vi "Lab Panel V5.24.1.vi"() -> ()   [LabVIEW 2013] (continued)
                n852 = local write "run lab04-1"(w1517) -> ()
                n853 = case shown="True" w1517 {
                  tunnel: w1523 -> [_ w1561]
                  tunnel: w1522 -> [_ w1560]
                  tunnel: w1520 -> [w1525 w1559]
                  tunnel: w1521 -> [_ w1558]
                  tunnel: w1519 -> [_ w1557]
                  tunnel: [w1524 w1556] -> w1518
                  tunnel: w1516 -> [_ w1555]
                  tunnel: w1515 -> [_ w1554]
                  tunnel: w1514 -> [_ w1553]
                  tunnel: w1513 -> [_ w1551]
                  frame False {
                    # "stop test"
                    n854 = stacked-sequence {
                      tunnel: w1525 -> [w1534 _]
                      tunnel: [w1526 _] -> w1524
                      frame #0 {
                        n855 = local read "DISP LAB04-1"() -> (w1533:T4)
                        n856 = Unbundle(w1533) -> ("CYCLE"=w1531:dbl, "MINS"=w1532:dbl)  [unwired: 1 out]
                        n857 = case shown="\"CYCLE TEST\"" w1534 {
                          tunnel: w1532 -> [_ _ w1541]
                          tunnel: w1531 -> [w1539 w1540 _]
                          tunnel: [w1539 w1540 w1541] -> w1530
                          frame "CHART TEST", Default {
                          }
                          frame "CYCLE TEST" {
                          }
                          frame "T-RISE TEST" {
                          }
                        }
                        n858 = local read "TDMS LAB04-1"() -> (w1538:refnum<k34>)
                        n859 = Build Array("STOPPED") -> (w1535:string[])
                        n860 = Build Array(w1530) -> (w1529:dbl[])
                        n861 = TDMS Write(0:w1538, 5:"TEST RESULT", 7:w1535, 9:w1529) -> (4:w1527:refnum<k34>, 15:w1528:errorcluster)  [unwired: 2 in, 2 out]
                        n862 = TDMS Close(8:w1528, 11:w1527) -> (0:w1526:errorcluster)  [unwired: 1 out]
                      }
                      frame #1 {
                        n863 = local read "DISP LAB04-1"() -> (w1545:T4)
                        n864 = stacked-sequence {
                          tunnel: "LAB04-1" -> [w1547 w1549]
                          frame #0 {
                            n865 = call "sub vi - defrag tdms v1.vi"("panel id"=w1547) -> ("error out"=w1546:errorcluster)  [unwired: 10 in]
                            n866 = local write "data file error"(w1546) -> ()
                          }
                          frame #1 {
                            n867 = call "Save data file (stop) v3.vi"("panel id"=w1549) -> ("network file save error"=w1548:errorcluster)  [unwired: 9 in, 1 out]
                            n868 = local write "RESULT LAB04-1"(FALSE) -> ()
                            n869 = local write "data file error"(w1548) -> ()
                          }
                        }
                        n870 = Bundle(cluster=w1545, "STATUS"="STOP") -> (w1543:T4)  [unwired: 2 in]
                        n871 = local write "DISP LAB04-1"(w1543) -> ()
                      }
                    }
                  }
                  frame True {
                    n872 = local read "SIG LAB04-1"() -> (w1552:T2)
                    n873 = stacked-sequence {
                      seq-local: [w1563 _] -> [_ w1567]
                      tunnel: w1561 -> [_ w1577]
                      tunnel: w1560 -> [_ w1576]
                      tunnel: w1559 -> [_ w1575]
                      tunnel: w1558 -> [_ w1574]
                      tunnel: w1557 -> [_ w1573]
                      tunnel: [_ w1572] -> w1556
                      tunnel: w1555 -> [_ w1571]
                      tunnel: w1554 -> [_ w1570]
                      tunnel: w1553 -> [_ w1569]
                      tunnel: w1552 -> [w1562 w1568]
                      tunnel: w1551 -> [_ w1566]
                      frame #0 {
                        n874 = Unbundle(w1562) -> ("AMPS"=w1565:dbl)  [unwired: 4 out]
                        n875 = call "Check For Amps on v1.vi"("ID"="LAB04-1", "amps"=w1565) -> ("amps"=w1563:bool)  [unwired: 9 in]
                      }
                      frame #1 {
                        n876 = case shown="True" w1567 {
                          tunnel: w1577 -> [_ w1590]
                          tunnel: w1576 -> [_ w1589]
                          tunnel: w1575 -> [_ w1588]
                          tunnel: w1574 -> [_ w1587]
                          tunnel: w1573 -> [_ w1586]
                          tunnel: [errorcluster {"status"=FALSE, "code"=0, "source"=""} ("error out") w1585] -> w1572
                          tunnel: w1571 -> [_ w1584]
                          tunnel: w1570 -> [_ w1583]
                          tunnel: w1569 -> [_ w1582]
                          tunnel: w1568 -> [_ w1581]
                          tunnel: w1566 -> [_ w1580]
                          frame False {
                            w1578 = FALSE
                            n877 = local write "RUN LAB04-1"(w1578) -> ()
                            n878 = local write "run lab04-1"(w1578) -> ()
                          }
                          frame True {
                            n879 = stacked-sequence {
                              seq-local: [w1591 _ _ _ _] -> [_ w1615 _ _ _]
                              tunnel: w1590 -> [w1596 _ _ _ _]
                              tunnel: w1589 -> [w1592 _ _ _ _]
                              tunnel: w1588 -> [w1606 _ _ _ _]
                              tunnel: w1587 -> [w1599 _ _ _ _]
                              tunnel: w1586 -> [w1594 _ _ _ _]
                              tunnel: [_ w1610 _ _ _] -> w1585
                              tunnel: w1584 -> [_ _ _ w1636 _]
                              tunnel: w1583 -> [_ _ _ w1635 _]
                              tunnel: w1582 -> [_ _ _ w1634 _]
                              tunnel: w1581 -> [_ _ _ _ _]
                              tunnel: w1580 -> [_ _ _ _ w1650]
                              frame #0 {
                                w1593 = "\\"
                                n880 = local read "SET LAB04-1"() -> (w1601:T5)
                                n881 = case shown="\"CYCLE TEST\"" w1606 {
                                tunnel: ["L04-1-CHART TEST-" "L04-1-CYCLE TEST-" "L04-1-T-RISE TEST-"] -> w1602
                                frame "CHART TEST", Default {
                                }
                                frame "CYCLE TEST" {
                                }
                                frame "T-RISE TEST" {
                                }
                                }
                                n882 = Unbundle(w1601) -> ("DESCRIPTION"=w1600:string)  [unwired: 4 out]
                                n883 = Concatenate Strings(w1596, "\\", w1594, w1593, w1592, w1593) -> (w1603:string)
                                n884 = String To Path(string=w1603) -> (path=w1605:path)
                                n885 = Concatenate Strings(w1603, w1602, w1600, "-", w1599, ".tdms") -> (w1591:string)
                                n886 = Create Folder(path (use dialog)=w1605) -> (error out=w1604:errorcluster)  [unwired: 2 in, 2 out]
                                n887 = global write "Global 1.vi" "LAB04-1 FILE"(w1591) -> ()
                                n888 = call <vilib>:"Clear Errors.vi"("error in (no error)"=w1604) -> ()  [unwired: 6 in, 1 out]
                              }
                              frame #1 {
                                (unwired) FALSE
                                n889 = String To Path(string=w1615) -> (path=w1611:path)
                                n890 = TDMS Open(6:FALSE, 10:T21."create or replace" ("operation (0:open)"), 11:w1611) -> (0:w1610:errorcluster, 3:→"TDMS LAB04-1":refnum<k34>)  [unwired: 4 in]
                              }
                              frame #2 {
                                n891 = local read "SET LAB04-1"() -> (w1621:T5)
                                n892 = local read "TDMS LAB04-1"() -> (w1632:refnum<k34>)
                                n893 = Build Array("Testers Name", "Description", "Set Test Cycles", "T-Rise minutes", "T-Rise Deg C") -> (w1622:string[])
                                n894 = Unbundle(w1621) -> ("NAME"=w1620:string, "DESCRIPTION"=w1619:string, "CYCLES"=w1618:dbl, "T-RISE mins"=w1617:dbl, "T-RISE deg C"=w1616:dbl)
                                n895 = Number To Decimal String(number=w1618) -> (decimal integer string=w1631:string)  [unwired: 1 in]
                                n896 = Number To Decimal String(number=w1617) -> (decimal integer string=w1630:string)  [unwired: 1 in]
                                n897 = Number To Decimal String(number=w1616) -> (decimal integer string=w1629:string)  [unwired: 1 in]
                                n898 = Build Array(w1620, w1619, w1631, w1630, w1629) -> (w1628:string[])
                                n899 = TDMS Set Properties(5:w1628, 7:w1622, 11:w1632) -> ()  [unwired: 3 in, 4 out]
                              }
                              frame #3 {
                                n900 = local read "DISP LAB04-1"() -> (w1637:T4)
                                n901 = Concatenate Strings("LAB04-1  ", w1636) -> (w1638:string)
                                n902 = Two Button Dialog(message=w1638, 1:w1634, 2:w1635) -> (T button?=w1640:bool)
                                n903 = case shown="True" w1640 {
                                tunnel: w1637 -> [w1647 w1648]
                                tunnel: [w1647 w1648] -> w1644
                                tunnel: [w1646 w1649] -> w1643
                                tunnel: [w1645 w1649] -> w1642
                                frame False {
                                n904 = Unbundle(w1647) -> ("CYCLE"=w1646:dbl, "MINS"=w1645:dbl)  [unwired: 1 out]
                                }
                                frame True {
                                w1649 = 0.0
                                }
                                }
                                n905 = Bundle(cluster=w1644, "CYCLE"=w1643, "MINS"=w1642, "STATUS"="RUN") -> (w1633:T4)
                                n906 = local write "DISP LAB04-1"(w1633) -> ()
                              }
                              frame #4 {
                                n907 = local read "TEMP START LAB04-1"() -> (w1652:cluster{"TL":dbl, "TN":dbl})
                                n908 = Bundle(cluster=w1652, "TL"=w1650, "TN"=w1650) -> (w1651:cluster{"TL":dbl, "TN":dbl})
                                n909 = local write "TEMP START LAB04-1"(w1651) -> ()
                              }
                            }
                          }
                        }
                      }
                    }
                  }
                }
              }
              event "RUN LAB04-2": Value Change {
                n910 = event-data() -> ("NewVal"=w1657:bool)  [unwired: 1 in, 5 out]
                n911 = local write "run lab04-2"(w1657) -> ()
                n912 = case shown="True" w1657 {
                  tunnel: w1663 -> [_ w1701]
                  tunnel: w1662 -> [_ w1700]
                  tunnel: w1660 -> [w1665 w1699]
                  tunnel: w1661 -> [_ w1698]
                  tunnel: w1659 -> [_ w1697]
                  tunnel: [w1664 w1696] -> w1658
                  tunnel: w1656 -> [_ w1695]
                  tunnel: w1655 -> [_ w1694]
                  tunnel: w1654 -> [_ w1693]
                  tunnel: w1653 -> [_ w1691]
                  frame False {
                    # "stop test"
                    n913 = stacked-sequence {
                      tunnel: w1665 -> [w1674 _]
                      tunnel: [w1666 _] -> w1664
                      frame #0 {
                        n914 = local read "DISP LAB04-2"() -> (w1673:T4)
                        n915 = Unbundle(w1673) -> ("CYCLE"=w1671:dbl, "MINS"=w1672:dbl)  [unwired: 1 out]
                        n916 = case shown="\"CYCLE TEST\"" w1674 {
                          tunnel: w1672 -> [_ _ w1681]
                          tunnel: w1671 -> [w1679 w1680 _]
                          tunnel: [w1679 w1680 w1681] -> w1670
                          frame "CHART TEST", Default {
                          }
                          frame "CYCLE TEST" {
                          }
                          frame "T-RISE TEST" {
                          }
                        }
                        n917 = local read "TDMS LAB04-2"() -> (w1678:refnum<k34>)
                        n918 = Build Array("STOPPED") -> (w1675:string[])
                        n919 = Build Array(w1670) -> (w1669:dbl[])
                        n920 = TDMS Write(0:w1678, 5:"TEST RESULT", 7:w1675, 9:w1669) -> (4:w1667:refnum<k34>, 15:w1668:errorcluster)  [unwired: 2 in, 2 out]
                        n921 = TDMS Close(8:w1668, 11:w1667) -> (0:w1666:errorcluster)  [unwired: 1 out]
                      }
                      frame #1 {
                        n922 = local read "DISP LAB04-2"() -> (w1685:T4)
                        n923 = stacked-sequence {
                          tunnel: "LAB04-2" -> [w1687 w1689]
                          frame #0 {
                            n924 = call "sub vi - defrag tdms v1.vi"("panel id"=w1687) -> ("error out"=w1686:errorcluster)  [unwired: 10 in]
                            n925 = local write "data file error"(w1686) -> ()
                          }
                          frame #1 {
                            n926 = call "Save data file (stop) v3.vi"("panel id"=w1689) -> ("network file save error"=w1688:errorcluster)  [unwired: 9 in, 1 out]
                            n927 = local write "RESULT LAB04-2"(FALSE) -> ()
                            n928 = local write "data file error"(w1688) -> ()
                          }
                        }
                        n929 = Bundle(cluster=w1685, "STATUS"="STOP") -> (w1683:T4)  [unwired: 2 in]
                        n930 = local write "DISP LAB04-2"(w1683) -> ()
                      }
                    }
                  }
                  frame True {
                    n931 = local read "SIG LAB04-2"() -> (w1692:T2)
                    n932 = stacked-sequence {
                      seq-local: [w1703 _] -> [_ w1707]
                      tunnel: w1701 -> [_ w1717]
                      tunnel: w1700 -> [_ w1716]
                      tunnel: w1699 -> [_ w1715]
                      tunnel: w1698 -> [_ w1714]
                      tunnel: w1697 -> [_ w1713]
                      tunnel: [_ w1712] -> w1696
                      tunnel: w1695 -> [_ w1711]
                      tunnel: w1694 -> [_ w1710]
                      tunnel: w1693 -> [_ w1709]
                      tunnel: w1692 -> [w1702 w1708]
                      tunnel: w1691 -> [_ w1706]
                      frame #0 {
                        n933 = Unbundle(w1702) -> ("AMPS"=w1705:dbl)  [unwired: 4 out]
                        n934 = call "Check For Amps on v1.vi"("ID"="LAB04-2", "amps"=w1705) -> ("amps"=w1703:bool)  [unwired: 9 in]
                      }
                      frame #1 {
                        n935 = case shown="True" w1707 {
                          tunnel: w1717 -> [_ w1730]
                          tunnel: w1716 -> [_ w1729]
                          tunnel: w1715 -> [_ w1728]
                          tunnel: w1714 -> [_ w1727]
                          tunnel: w1713 -> [_ w1726]
                          tunnel: [errorcluster {"status"=FALSE, "code"=0, "source"=""} ("error out") w1725] -> w1712
                          tunnel: w1711 -> [_ w1724]
                          tunnel: w1710 -> [_ w1723]
                          tunnel: w1709 -> [_ w1722]
                          tunnel: w1708 -> [_ w1721]
                          tunnel: w1706 -> [_ w1720]
                          frame False {
                            w1718 = FALSE
                            n936 = local write "RUN LAB04-2"(w1718) -> ()
                            n937 = local write "run lab04-2"(w1718) -> ()
                          }
                          frame True {
                            n938 = stacked-sequence {
                              seq-local: [w1731 _ _ _ _] -> [_ w1755 _ _ _]
                              tunnel: w1730 -> [w1736 _ _ _ _]
                              tunnel: w1729 -> [w1732 _ _ _ _]
                              tunnel: w1728 -> [w1746 _ _ _ _]
                              tunnel: w1727 -> [w1739 _ _ _ _]
                              tunnel: w1726 -> [w1734 _ _ _ _]
                              tunnel: [_ w1750 _ _ _] -> w1725
                              tunnel: w1724 -> [_ _ _ w1776 _]
                              tunnel: w1723 -> [_ _ _ w1775 _]
                              tunnel: w1722 -> [_ _ _ w1774 _]
                              tunnel: w1721 -> [_ _ _ _ _]
                              tunnel: w1720 -> [_ _ _ _ w1790]
                              frame #0 {
                                w1733 = "\\"
                                n939 = local read "SET LAB04-2"() -> (w1741:T5)
                                n940 = case shown="\"CHART TEST\", Default" w1746 {
                                tunnel: ["L04-2-CHART TEST-" "L04-2-CYCLE TEST-" "L04-2-T-RISE TEST-"] -> w1742
                                frame "CHART TEST", Default {
                                }
                                frame "CYCLE TEST" {
                                }
                                frame "T-RISE TEST" {
                                }
                                }
                                n941 = Unbundle(w1741) -> ("DESCRIPTION"=w1740:string)  [unwired: 4 out]
                                n942 = Concatenate Strings(w1736, "\\", w1734, w1733, w1732, w1733) -> (w1743:string)
                                n943 = String To Path(string=w1743) -> (path=w1745:path)
                                n944 = Concatenate Strings(w1743, w1742, w1740, "-", w1739, ".tdms") -> (w1731:string)
                                n945 = Create Folder(path (use dialog)=w1745) -> (error out=w1744:errorcluster)  [unwired: 2 in, 2 out]
                                n946 = global write "Global 1.vi" "LAB04-2 FILE"(w1731) -> ()
                                n947 = call <vilib>:"Clear Errors.vi"("error in (no error)"=w1744) -> ()  [unwired: 6 in, 1 out]
                              }
                              frame #1 {
                                (unwired) FALSE
                                n948 = String To Path(string=w1755) -> (path=w1751:path)
                                n949 = TDMS Open(6:FALSE, 10:T21."create or replace" ("operation (0:open)"), 11:w1751) -> (0:w1750:errorcluster, 3:→"TDMS LAB04-2":refnum<k34>)  [unwired: 4 in]
                              }
                              frame #2 {
                                n950 = local read "SET LAB04-2"() -> (w1761:T5)
                                n951 = local read "TDMS LAB04-2"() -> (w1772:refnum<k34>)
                                n952 = Build Array("Testers Name", "Description", "Set Test Cycles", "T-Rise minutes", "T-Rise Deg C") -> (w1762:string[])
                                n953 = Unbundle(w1761) -> ("NAME"=w1760:string, "DESCRIPTION"=w1759:string, "CYCLES"=w1758:dbl, "T-RISE mins"=w1757:dbl, "T-RISE deg C"=w1756:dbl)
                                n954 = Number To Decimal String(number=w1758) -> (decimal integer string=w1771:string)  [unwired: 1 in]
                                n955 = Number To Decimal String(number=w1757) -> (decimal integer string=w1770:string)  [unwired: 1 in]
                                n956 = Number To Decimal String(number=w1756) -> (decimal integer string=w1769:string)  [unwired: 1 in]
                                n957 = Build Array(w1760, w1759, w1771, w1770, w1769) -> (w1768:string[])
                                n958 = TDMS Set Properties(5:w1768, 7:w1762, 11:w1772) -> ()  [unwired: 3 in, 4 out]
                              }
                              frame #3 {
                                n959 = local read "DISP LAB04-2"() -> (w1777:T4)
                                n960 = Concatenate Strings("LAB04-2 ", w1776) -> (w1778:string)
                                n961 = Two Button Dialog(message=w1778, 1:w1774, 2:w1775) -> (T button?=w1780:bool)
                                n962 = case shown="True" w1780 {
                                tunnel: w1777 -> [w1787 w1788]
                                tunnel: [w1787 w1788] -> w1784
                                tunnel: [w1786 w1789] -> w1783
                                tunnel: [w1785 w1789] -> w1782
                                frame False {
                                n963 = Unbundle(w1787) -> ("CYCLE"=w1786:dbl, "MINS"=w1785:dbl)  [unwired: 1 out]
                                }
                                frame True {
                                w1789 = 0.0
                                }
                                }
                                n964 = Bundle(cluster=w1784, "CYCLE"=w1783, "MINS"=w1782, "STATUS"="RUN") -> (w1773:T4)
                                n965 = local write "DISP LAB04-2"(w1773) -> ()
                              }
                              frame #4 {
                                n966 = local read "TEMP START LAB04-2"() -> (w1792:cluster{"TL":dbl, "TN":dbl})
                                n967 = Bundle(cluster=w1792, "TL"=w1790, "TN"=w1790) -> (w1791:cluster{"TL":dbl, "TN":dbl})
                                n968 = local write "TEMP START LAB04-2"(w1791) -> ()
                              }
                            }
                          }
                        }
                      }
                    }
                  }
                }
              }
              event "RUN LAB05-1": Value Change {
                n969 = event-data() -> ("NewVal"=w1797:bool)  [unwired: 1 in, 5 out]
                n970 = local write "run lab05-1"(w1797) -> ()
                n971 = case shown="True" w1797 {
                  tunnel: w1803 -> [_ w1841]
                  tunnel: w1802 -> [_ w1840]
                  tunnel: w1800 -> [w1805 w1839]
                  tunnel: w1801 -> [_ w1838]
                  tunnel: w1799 -> [_ w1837]
                  tunnel: [w1804 w1836] -> w1798
                  tunnel: w1796 -> [_ w1835]
                  tunnel: w1795 -> [_ w1834]
                  tunnel: w1794 -> [_ w1833]
                  tunnel: w1793 -> [_ w1831]
                  frame False {
                    # "stop test"
                    n972 = stacked-sequence {
                      tunnel: w1805 -> [w1814 _]
                      tunnel: [w1806 _] -> w1804
                      frame #0 {
                        n973 = local read "DISP LAB05-1"() -> (w1813:T4)
                        n974 = Unbundle(w1813) -> ("CYCLE"=w1811:dbl, "MINS"=w1812:dbl)  [unwired: 1 out]
                        n975 = case shown="\"CYCLE TEST\"" w1814 {
                          tunnel: w1812 -> [_ _ w1821]
                          tunnel: w1811 -> [w1819 w1820 _]
                          tunnel: [w1819 w1820 w1821] -> w1810
                          frame "CHART TEST", Default {
                          }
                          frame "CYCLE TEST" {
                          }
                          frame "T-RISE TEST" {
                          }
                        }
                        n976 = local read "TDMS LAB05-1"() -> (w1818:refnum<k34>)
                        n977 = Build Array("STOPPED") -> (w1815:string[])
                        n978 = Build Array(w1810) -> (w1809:dbl[])
                        n979 = TDMS Write(0:w1818, 5:"TEST RESULT", 7:w1815, 9:w1809) -> (4:w1807:refnum<k34>, 15:w1808:errorcluster)  [unwired: 2 in, 2 out]
                        n980 = TDMS Close(8:w1808, 11:w1807) -> (0:w1806:errorcluster)  [unwired: 1 out]
                      }
                      frame #1 {
                        n981 = local read "DISP LAB05-1"() -> (w1825:T4)
                        n982 = stacked-sequence {
                          tunnel: "LAB05-1" -> [w1827 w1829]
                          frame #0 {
                            n983 = call "sub vi - defrag tdms v1.vi"("panel id"=w1827) -> ("error out"=w1826:errorcluster)  [unwired: 10 in]
                            n984 = local write "data file error"(w1826) -> ()
                          }
                          frame #1 {
                            n985 = call "Save data file (stop) v3.vi"("panel id"=w1829) -> ("network file save error"=w1828:errorcluster)  [unwired: 9 in, 1 out]
                            n986 = local write "RESULT LAB05-1"(FALSE) -> ()
                            n987 = local write "data file error"(w1828) -> ()
                          }
                        }
                        n988 = Bundle(cluster=w1825, "STATUS"="STOP") -> (w1823:T4)  [unwired: 2 in]
                        n989 = local write "DISP LAB05-1"(w1823) -> ()
                      }
                    }
                  }
                  frame True {
                    n990 = local read "SIG LAB05-1"() -> (w1832:T2)
                    n991 = stacked-sequence {
                      seq-local: [w1843 _] -> [_ w1847]
                      tunnel: w1841 -> [_ w1857]
                      tunnel: w1840 -> [_ w1856]
                      tunnel: w1839 -> [_ w1855]
                      tunnel: w1838 -> [_ w1854]
                      tunnel: w1837 -> [_ w1853]
                      tunnel: [_ w1852] -> w1836
                      tunnel: w1835 -> [_ w1851]
                      tunnel: w1834 -> [_ w1850]
                      tunnel: w1833 -> [_ w1849]
                      tunnel: w1832 -> [w1842 w1848]
                      tunnel: w1831 -> [_ w1846]
                      frame #0 {
                        n992 = Unbundle(w1842) -> ("AMPS"=w1845:dbl)  [unwired: 4 out]
                        n993 = call "Check For Amps on v1.vi"("ID"="LAB05-1", "amps"=w1845) -> ("amps"=w1843:bool)  [unwired: 9 in]
                      }
                      frame #1 {
                        n994 = case shown="True" w1847 {
                          tunnel: w1857 -> [_ w1870]
                          tunnel: w1856 -> [_ w1869]
                          tunnel: w1855 -> [_ w1868]
                          tunnel: w1854 -> [_ w1867]
                          tunnel: w1853 -> [_ w1866]
                          tunnel: [errorcluster {"status"=FALSE, "code"=0, "source"=""} ("error out") w1865] -> w1852
                          tunnel: w1851 -> [_ w1864]
                          tunnel: w1850 -> [_ w1863]
                          tunnel: w1849 -> [_ w1862]
                          tunnel: w1848 -> [_ w1861]
                          tunnel: w1846 -> [_ w1860]
                          frame False {
                            w1858 = FALSE
                            n995 = local write "RUN LAB05-1"(w1858) -> ()
                            n996 = local write "run lab05-1"(w1858) -> ()
                          }
                          frame True {
                            n997 = stacked-sequence {
                              seq-local: [w1871 _ _ _ _] -> [_ w1895 _ _ _]
                              tunnel: w1870 -> [w1876 _ _ _ _]
                              tunnel: w1869 -> [w1872 _ _ _ _]
                              tunnel: w1868 -> [w1886 _ _ _ _]
                              tunnel: w1867 -> [w1879 _ _ _ _]
                              tunnel: w1866 -> [w1874 _ _ _ _]
                              tunnel: [_ w1890 _ _ _] -> w1865
                              tunnel: w1864 -> [_ _ _ w1915 _]
                              tunnel: w1863 -> [_ _ _ w1914 _]
                              tunnel: w1862 -> [_ _ _ w1913 _]
                              tunnel: w1861 -> [_ _ _ _ _]
                              tunnel: w1860 -> [_ _ _ _ w1930]
                              frame #0 {
                                w1873 = "\\"
                                n998 = local read "SET LAB05-1"() -> (w1881:T5)
                                n999 = case shown="\"CYCLE TEST\"" w1886 {
                                tunnel: ["L05-1-CHART TEST-" "L05-1-CYCLE TEST-" "L05-1-T-RISE TEST-"] -> w1882
                                frame "CHART TEST", Default {
                                }
                                frame "CYCLE TEST" {
                                }
                                frame "T-RISE TEST" {
                                }
                                }
                                n1000 = Unbundle(w1881) -> ("DESCRIPTION"=w1880:string)  [unwired: 4 out]
                                n1001 = Concatenate Strings(w1876, "\\", w1874, w1873, w1872, w1873) -> (w1883:string)
                                n1002 = String To Path(string=w1883) -> (path=w1885:path)
                                n1003 = Concatenate Strings(w1883, w1882, w1880, "-", w1879, ".tdms") -> (w1871:string)
                                n1004 = Create Folder(path (use dialog)=w1885) -> (error out=w1884:errorcluster)  [unwired: 2 in, 2 out]
                                n1005 = global write "Global 1.vi" "LAB05-1 FILE"(w1871) -> ()
                                n1006 = call <vilib>:"Clear Errors.vi"("error in (no error)"=w1884) -> ()  [unwired: 6 in, 1 out]
                              }
                              frame #1 {
                                (unwired) FALSE
                                n1007 = String To Path(string=w1895) -> (path=w1891:path)
                                n1008 = TDMS Open(6:FALSE, 10:T21."create or replace" ("operation (0:open)"), 11:w1891) -> (0:w1890:errorcluster, 3:→"TDMS LAB05-1":refnum<k34>)  [unwired: 4 in]
                              }
                              frame #2 {
                                n1009 = local read "SET LAB05-1"() -> (w1901:T5)
                                n1010 = local read "TDMS LAB05-1"() -> (w1912:refnum<k34>)
                                n1011 = Build Array("Testers Name", "Description", "Set Test Cycles", "T-Rise minutes", "T-Rise Deg C") -> (w1902:string[])
                                n1012 = Unbundle(w1901) -> ("NAME"=w1900:string, "DESCRIPTION"=w1899:string, "CYCLES"=w1898:dbl, "T-RISE mins"=w1897:dbl, "T-RISE deg C"=w1896:dbl)
                                n1013 = Number To Decimal String(number=w1898) -> (decimal integer string=w1911:string)  [unwired: 1 in]
                                n1014 = Number To Decimal String(number=w1897) -> (decimal integer string=w1910:string)  [unwired: 1 in]
                                n1015 = Number To Decimal String(number=w1896) -> (decimal integer string=w1909:string)  [unwired: 1 in]
                                n1016 = Build Array(w1900, w1899, w1911, w1910, w1909) -> (w1908:string[])
                                n1017 = TDMS Set Properties(5:w1908, 7:w1902, 11:w1912) -> ()  [unwired: 3 in, 4 out]
                              }
                              frame #3 {
                                n1018 = local read "DISP LAB05-1"() -> (w1917:T4)
                                n1019 = Concatenate Strings("LAB05-1  ", w1915) -> (w1918:string)
                                n1020 = Two Button Dialog(message=w1918, 1:w1913, 2:w1914) -> (T button?=w1920:bool)
                                n1021 = case shown="True" w1920 {
                                tunnel: w1917 -> [w1927 w1928]
                                tunnel: [w1927 w1928] -> w1924
                                tunnel: [w1926 w1929] -> w1923
                                tunnel: [w1925 w1929] -> w1922
                                frame False {
                                n1022 = Unbundle(w1927) -> ("CYCLE"=w1926:dbl, "MINS"=w1925:dbl)  [unwired: 1 out]
                                }
                                frame True {
                                w1929 = 0.0
                                }
                                }
                                n1023 = Bundle(cluster=w1924, "CYCLE"=w1923, "MINS"=w1922, "STATUS"="RUN") -> (w1916:T4)
                                n1024 = local write "DISP LAB05-1"(w1916) -> ()
                              }
                              frame #4 {
                                n1025 = local read "TEMP START LAB05-1"() -> (w1932:cluster{"TL":dbl, "TN":dbl})
                                n1026 = Bundle(cluster=w1932, "TL"=w1930, "TN"=w1930) -> (w1931:cluster{"TL":dbl, "TN":dbl})
                                n1027 = local write "TEMP START LAB05-1"(w1931) -> ()
                              }
                            }
                          }
                        }
                      }
                    }
                  }
                }
              }
              event "RUN LAB05-2": Value Change {
                n1028 = event-data() -> ("NewVal"=w1938:bool)  [unwired: 1 in, 5 out]
                n1029 = local read "SIG LAB05-2"() -> (w1934:T2)
                n1030 = case shown="True" w1938 {
                  tunnel: w1944 -> [_ w1982]
                  tunnel: w1943 -> [_ w1981]
                  tunnel: w1941 -> [w1946 w1980]
                  tunnel: w1942 -> [_ w1979]
                  tunnel: w1940 -> [_ w1978]
                  tunnel: [w1945 w1977] -> w1939
                  tunnel: w1937 -> [_ w1976]
                  tunnel: w1936 -> [_ w1975]
                  tunnel: w1935 -> [_ w1974]
                  tunnel: w1934 -> [_ w1973]
                  tunnel: w1933 -> [_ w1972]
                  frame False {
                    # "stop test"
                    n1031 = stacked-sequence {
                      tunnel: w1946 -> [w1955 _]
                      tunnel: [w1947 _] -> w1945
                      frame #0 {
                        n1032 = local read "DISP LAB05-2"() -> (w1954:T4)
                        n1033 = Unbundle(w1954) -> ("CYCLE"=w1952:dbl, "MINS"=w1953:dbl)  [unwired: 1 out]
                        n1034 = case shown="\"CYCLE TEST\"" w1955 {
                          tunnel: w1953 -> [_ _ w1962]
                          tunnel: w1952 -> [w1960 w1961 _]
                          tunnel: [w1960 w1961 w1962] -> w1951
                          frame "CHART TEST", Default {
                          }
                          frame "CYCLE TEST" {
                          }
                          frame "T-RISE TEST" {
                          }
                        }
                        n1035 = local read "TDMS LAB05-2"() -> (w1959:refnum<k34>)
                        n1036 = Build Array("STOPPED") -> (w1956:string[])
                        n1037 = Build Array(w1951) -> (w1950:dbl[])
                        n1038 = TDMS Write(0:w1959, 5:"TEST RESULT", 7:w1956, 9:w1950) -> (4:w1948:refnum<k34>, 15:w1949:errorcluster)  [unwired: 2 in, 2 out]
                        n1039 = TDMS Close(8:w1949, 11:w1948) -> (0:w1947:errorcluster)  [unwired: 1 out]
                      }
                      frame #1 {
                        n1040 = local read "DISP LAB05-2"() -> (w1966:T4)
                        n1041 = stacked-sequence {
                          tunnel: "LAB05-2" -> [w1968 w1970]
                          frame #0 {
                            n1042 = call "sub vi - defrag tdms v1.vi"("panel id"=w1968) -> ("error out"=w1967:errorcluster)  [unwired: 10 in]
                            n1043 = local write "data file error"(w1967) -> ()
                          }
                          frame #1 {
                            n1044 = local write "RESULT LAB05-2"(FALSE) -> ()
                            n1045 = call "Save data file (stop) v3.vi"("panel id"=w1970) -> ("network file save error"=w1969:errorcluster)  [unwired: 9 in, 1 out]
                            n1046 = local write "data file error"(w1969) -> ()
                          }
                        }
                        n1047 = Bundle(cluster=w1966, "STATUS"="STOP") -> (w1964:T4)  [unwired: 2 in]
                        n1048 = local write "DISP LAB05-2"(w1964) -> ()
                      }
                    }
                  }
                  frame True {
                    n1049 = stacked-sequence {
                      seq-local: [w1984 _] -> [_ w1988]
                      tunnel: w1982 -> [_ w1998]
                      tunnel: w1981 -> [_ w1997]
                      tunnel: w1980 -> [_ w1996]
                      tunnel: w1979 -> [_ w1995]
                      tunnel: w1978 -> [_ w1994]
                      tunnel: [_ w1993] -> w1977
                      tunnel: w1976 -> [_ w1992]
                      tunnel: w1975 -> [_ w1991]
                      tunnel: w1974 -> [_ w1990]
                      tunnel: w1973 -> [w1983 w1989]
                      tunnel: w1972 -> [_ w1987]
                      frame #0 {
                        n1050 = Unbundle(w1983) -> ("AMPS"=w1986:dbl)  [unwired: 4 out]
                        n1051 = call "Check For Amps on v1.vi"("ID"="LAB05-2", "amps"=w1986) -> ("amps"=w1984:bool)  [unwired: 9 in]
                      }
                      frame #1 {
                        n1052 = case shown="True" w1988 {
                          tunnel: w1998 -> [_ w2011]
                          tunnel: w1997 -> [_ w2010]
                          tunnel: w1996 -> [_ w2009]
                          tunnel: w1995 -> [_ w2008]
                          tunnel: w1994 -> [_ w2007]
                          tunnel: [errorcluster {"status"=FALSE, "code"=0, "source"=""} ("error out") w2006] -> w1993
                          tunnel: w1992 -> [_ w2005]
                          tunnel: w1991 -> [_ w2004]
                          tunnel: w1990 -> [_ w2003]
                          tunnel: w1989 -> [_ w2002]
                          tunnel: w1987 -> [_ w2001]
                          frame False {
                            w1999 = FALSE
                            n1053 = local write "RUN LAB05-2"(w1999) -> ()
                            n1054 = local write "run lab05-2"(w1999) -> ()
                          }
                          frame True {
                            n1055 = stacked-sequence {
                              seq-local: [w2012 _ _ _ _] -> [_ w2036 _ _ _]
                              tunnel: w2011 -> [w2017 _ _ _ _]
                              tunnel: w2010 -> [w2013 _ _ _ _]
                              tunnel: w2009 -> [w2027 _ _ _ _]
                              tunnel: w2008 -> [w2020 _ _ _ _]
                              tunnel: w2007 -> [w2015 _ _ _ _]
                              tunnel: [_ w2031 _ _ _] -> w2006
                              tunnel: w2005 -> [_ _ _ w2056 _]
                              tunnel: w2004 -> [_ _ _ w2055 _]
                              tunnel: w2003 -> [_ _ _ w2054 _]
                              tunnel: w2002 -> [_ _ _ _ _]
                              tunnel: w2001 -> [_ _ _ _ w2071]
                              frame #0 {
                                w2014 = "\\"
                                n1056 = local read "SET LAB05-2"() -> (w2022:T5)
                                n1057 = case shown="\"CYCLE TEST\"" w2027 {
                                tunnel: ["L05-2-CHART TEST-" "L05-2-CYCLE TEST-" "L05-2-T-RISE TEST-"] -> w2023
                                frame "CHART TEST", Default {
                                }
                                frame "CYCLE TEST" {
                                }
                                frame "T-RISE TEST" {
                                }
                                }
                                n1058 = Unbundle(w2022) -> ("DESCRIPTION"=w2021:string)  [unwired: 4 out]
                                n1059 = Concatenate Strings(w2017, "\\", w2015, w2014, w2013, w2014) -> (w2024:string)
                                n1060 = String To Path(string=w2024) -> (path=w2026:path)
                                n1061 = Concatenate Strings(w2024, w2023, w2021, "-", w2020, ".tdms") -> (w2012:string)
                                n1062 = Create Folder(path (use dialog)=w2026) -> (error out=w2025:errorcluster)  [unwired: 2 in, 2 out]
                                n1063 = global write "Global 1.vi" "LAB05-2 FILE"(w2012) -> ()
                                n1064 = call <vilib>:"Clear Errors.vi"("error in (no error)"=w2025) -> ()  [unwired: 6 in, 1 out]
                              }
                              frame #1 {
                                (unwired) FALSE
                                n1065 = String To Path(string=w2036) -> (path=w2032:path)
                                n1066 = TDMS Open(6:FALSE, 10:T21."create or replace" ("operation (0:open)"), 11:w2032) -> (0:w2031:errorcluster, 3:→"TDMS LAB05-2":refnum<k34>)  [unwired: 4 in]
                              }
                              frame #2 {
                                n1067 = local read "SET LAB05-2"() -> (w2042:T5)
                                n1068 = local read "TDMS LAB05-2"() -> (w2053:refnum<k34>)
                                n1069 = Build Array("Testers Name", "Description", "Set Test Cycles", "T-Rise minutes", "T-Rise Deg C") -> (w2043:string[])
                                n1070 = Unbundle(w2042) -> ("NAME"=w2041:string, "DESCRIPTION"=w2040:string, "CYCLES"=w2039:dbl, "T-RISE mins"=w2038:dbl, "T-RISE deg C"=w2037:dbl)
                                n1071 = Number To Decimal String(number=w2039) -> (decimal integer string=w2052:string)  [unwired: 1 in]
                                n1072 = Number To Decimal String(number=w2038) -> (decimal integer string=w2051:string)  [unwired: 1 in]
                                n1073 = Number To Decimal String(number=w2037) -> (decimal integer string=w2050:string)  [unwired: 1 in]
                                n1074 = Build Array(w2041, w2040, w2052, w2051, w2050) -> (w2049:string[])
                                n1075 = TDMS Set Properties(5:w2049, 7:w2043, 11:w2053) -> ()  [unwired: 3 in, 4 out]
                              }
                              frame #3 {
                                n1076 = local read "DISP LAB05-2"() -> (w2058:T4)
                                n1077 = Concatenate Strings("LAB05-2  ", w2056) -> (w2059:string)
                                n1078 = Two Button Dialog(message=w2059, 1:w2054, 2:w2055) -> (T button?=w2061:bool)
                                n1079 = case shown="True" w2061 {
                                tunnel: w2058 -> [w2068 w2069]
                                tunnel: [w2068 w2069] -> w2065
                                tunnel: [w2067 w2070] -> w2064
                                tunnel: [w2066 w2070] -> w2063
                                frame False {
                                n1080 = Unbundle(w2068) -> ("CYCLE"=w2067:dbl, "MINS"=w2066:dbl)  [unwired: 1 out]
                                }
                                frame True {
                                w2070 = 0.0
                                }
                                }
                                n1081 = Bundle(cluster=w2065, "CYCLE"=w2064, "MINS"=w2063, "STATUS"="RUN") -> (w2057:T4)
                                n1082 = local write "DISP LAB05-2"(w2057) -> ()
                              }
                              frame #4 {
                                n1083 = local read "TEMP START LAB05-2"() -> (w2073:cluster{"TL":dbl, "TN":dbl})
                                n1084 = Bundle(cluster=w2073, "TL"=w2071, "TN"=w2071) -> (w2072:cluster{"TL":dbl, "TN":dbl})
                                n1085 = local write "TEMP START LAB05-2"(w2072) -> ()
                              }
                            }
                          }
                        }
                      }
                    }
                  }
                }
                n1086 = local write "run lab05-2"(w1938) -> ()
              }
            }
            n1087 = local write "data file error"(w642) -> ()
          }
          frame #4 {
            # "check if test cycles reached for cycle tests, if so then test pass"
            n1088 = stacked-sequence {
              tunnel: w2093 -> [_ _ _ _ _ _ _ _ _ _]
              tunnel: w2092 -> [_ _ _ _ _ _ _ _ _ _]
              tunnel: w2091 -> [_ _ _ _ _ _ _ _ _ _]
              tunnel: w2090 -> [_ _ _ _ _ _ _ _ _ _]
              tunnel: w2089 -> [_ _ _ _ _ _ _ _ _ _]
              tunnel: w2088 -> [_ _ _ _ _ _ _ _ _ _]
              tunnel: w2087 -> [_ _ _ _ _ _ _ _ _ _]
              tunnel: w2086 -> [_ _ _ _ _ _ _ _ _ _]
              tunnel: w2085 -> [_ _ _ _ _ _ _ _ _ _]
              tunnel: w2084 -> [_ _ _ _ _ _ _ _ _ _]
              tunnel: w2083 -> [w2099 _ _ _ _ _ _ _ _ _]
              tunnel: w2082 -> [_ w2134 _ _ _ _ _ _ _ _]
              tunnel: w2081 -> [_ _ w2174 _ _ _ _ _ _ _]
              tunnel: w2080 -> [_ _ _ w2214 _ _ _ _ _ _]
              tunnel: w2079 -> [_ _ _ _ w2254 _ _ _ _ _]
              tunnel: w2078 -> [_ _ _ _ _ w2294 _ _ _ _]
              tunnel: w2077 -> [_ _ _ _ _ _ w2334 _ _ _]
              tunnel: w2076 -> [_ _ _ _ _ _ _ w2374 _ _]
              tunnel: w2075 -> [_ _ _ _ _ _ _ _ w2414 _]
              tunnel: w2074 -> [_ _ _ _ _ _ _ _ _ w2454]
              frame #0 {
                # "LAB01-1"
                n1089 = Less?(x=w2099, y=2) -> (x < y?=w2097:bool)
                n1090 = local read "DISP LAB01-1"() -> (w2100:T4)
                n1091 = Unbundle(w2100) -> ("STATUS"=w2094:string)  [unwired: 2 out]
                n1092 = Equal?(x=w2094, y="RUN") -> (x = y?=w2096:bool)
                n1093 = And(x=w2096, y=w2097) -> (x .and. y?=w2095:bool)
                n1094 = case shown="True" w2095 {
                  tunnel: w2100 -> [_ w2105]
                  tunnel: w2099 -> [_ w2109]
                  frame False {
                  }
                  frame True {
                    n1095 = local read "SET LAB01-1"() -> (w2111:T5)
                    n1096 = local read "TDMS LAB01-1"() -> (w2104:refnum<k34>)
                    n1097 = Unbundle(w2111) -> ("CYCLES"=w2102:dbl, "T-RISE mins"=w2108:dbl)  [unwired: 3 out]
                    n1098 = case shown="\"CYCLE TEST\"" w2109 {
                      tunnel: w2108 -> [_ _ w2118]
                      tunnel: [w2113 w2115 w2118] -> w2107
                      tunnel: w2102 -> [w2113 w2115 _]
                      tunnel: ["CHART PASS" "CYCLE PASS" "T-RISE PASS"] -> w2106
                      frame "CHART TEST", Default {
                      }
                      frame "CYCLE TEST" {
                      }
                      frame "T-RISE TEST" {
                      }
                    }
                    n1099 = Unbundle(w2105) -> ("CYCLE"=w2110:dbl)  [unwired: 2 out]
                    n1100 = Increment(x=w2102) -> (x+1=w2103:dbl)
                    n1101 = Greater Or Equal?(x=w2110, y=w2103) -> (x >= y?=w2112:bool)
                    n1102 = case shown="True" w2112 {
                      tunnel: w2107 -> [w2122 _]
                      tunnel: w2106 -> [w2121 _]
                      tunnel: w2105 -> [w2120 _]
                      tunnel: w2104 -> [w2119 _]
                      frame True {
                        n1103 = stacked-sequence {
                          tunnel: w2122 -> [w2126 _]
                          tunnel: w2121 -> [w2124 w2130]
                          tunnel: w2120 -> [_ w2133]
                          tunnel: w2119 -> [w2123 _]
                          frame #0 {
                            n1104 = Build Array(w2124) -> (w2127:string[])
                            n1105 = Build Array(w2126) -> (w2125:dbl[])
                            n1106 = TDMS Write(0:w2123, 5:"TEST PASS", 7:w2127, 9:w2125) -> (15:w2129:errorcluster)  [unwired: 2 in, 3 out]
                            n1107 = local write "data file error"(w2129) -> ()
                          }
                          frame #1 {
                            n1108 = Bundle(cluster=w2133, "STATUS"=w2130) -> (w2131:T4)  [unwired: 2 in]
                            n1109 = local write "RESULT LAB01-1"(TRUE) -> ()
                            n1110 = local write "DISP LAB01-1"(w2131) -> ()
                          }
                        }
                      }
                      frame False {
                      }
                    }
                  }
                }
              }
              frame #1 {
                # "LAB01-2"
                n1111 = Less?(x=w2134, y=2) -> (x < y?=w2137:bool)
                n1112 = local read "DISP LAB01-2"() -> (w2139:T4)
                n1113 = Unbundle(w2139) -> ("STATUS"=w2140:string)  [unwired: 2 out]
                n1114 = Equal?(x=w2140, y="RUN") -> (x = y?=w2136:bool)
                n1115 = And(x=w2136, y=w2137) -> (x .and. y?=w2135:bool)
                n1116 = case shown="True" w2135 {
                  tunnel: w2139 -> [_ w2145]
                  tunnel: w2134 -> [_ w2149]
                  frame False {
                  }
                  frame True {
                    n1117 = local read "SET LAB01-2"() -> (w2151:T5)
                    n1118 = local read "TDMS LAB01-2"() -> (w2144:refnum<k34>)
                    n1119 = Unbundle(w2151) -> ("CYCLES"=w2142:dbl, "T-RISE mins"=w2148:dbl)  [unwired: 3 out]
                    n1120 = case shown="\"T-RISE TEST\"" w2149 {
                      tunnel: w2148 -> [_ _ w2158]
                      tunnel: [w2153 w2155 w2158] -> w2147
                      tunnel: w2142 -> [w2153 w2155 _]
                      tunnel: ["CHART PASS" "CYCLE PASS" "T-RISE PASS"] -> w2146
                      frame "CHART TEST", Default {
                      }
                      frame "CYCLE TEST" {
                      }
                      frame "T-RISE TEST" {
                      }
                    }
                    n1121 = Unbundle(w2145) -> ("CYCLE"=w2150:dbl)  [unwired: 2 out]
                    n1122 = Increment(x=w2142) -> (x+1=w2143:dbl)
                    n1123 = Greater Or Equal?(x=w2150, y=w2143) -> (x >= y?=w2152:bool)
                    n1124 = case shown="True" w2152 {
                      tunnel: w2147 -> [w2162 _]
